vi "Step 2.vi"(8 "error in (no error)":errorcluster, 11 "HeatUp Data in":string[][](array[string])) -> (0 "error out":errorcluster, 1 "Large Draw":dbl[][](graph), 2 "Draw Flag":string[][](array[string]), 3 "Large Draw Flag Gallons":dbl)   [LabVIEW 2016]
uses:
  <vilib>/Utility/error.llb/DialogType.ctl
panel:
  out "Time":dbl
  # "Data with Stripped Header"
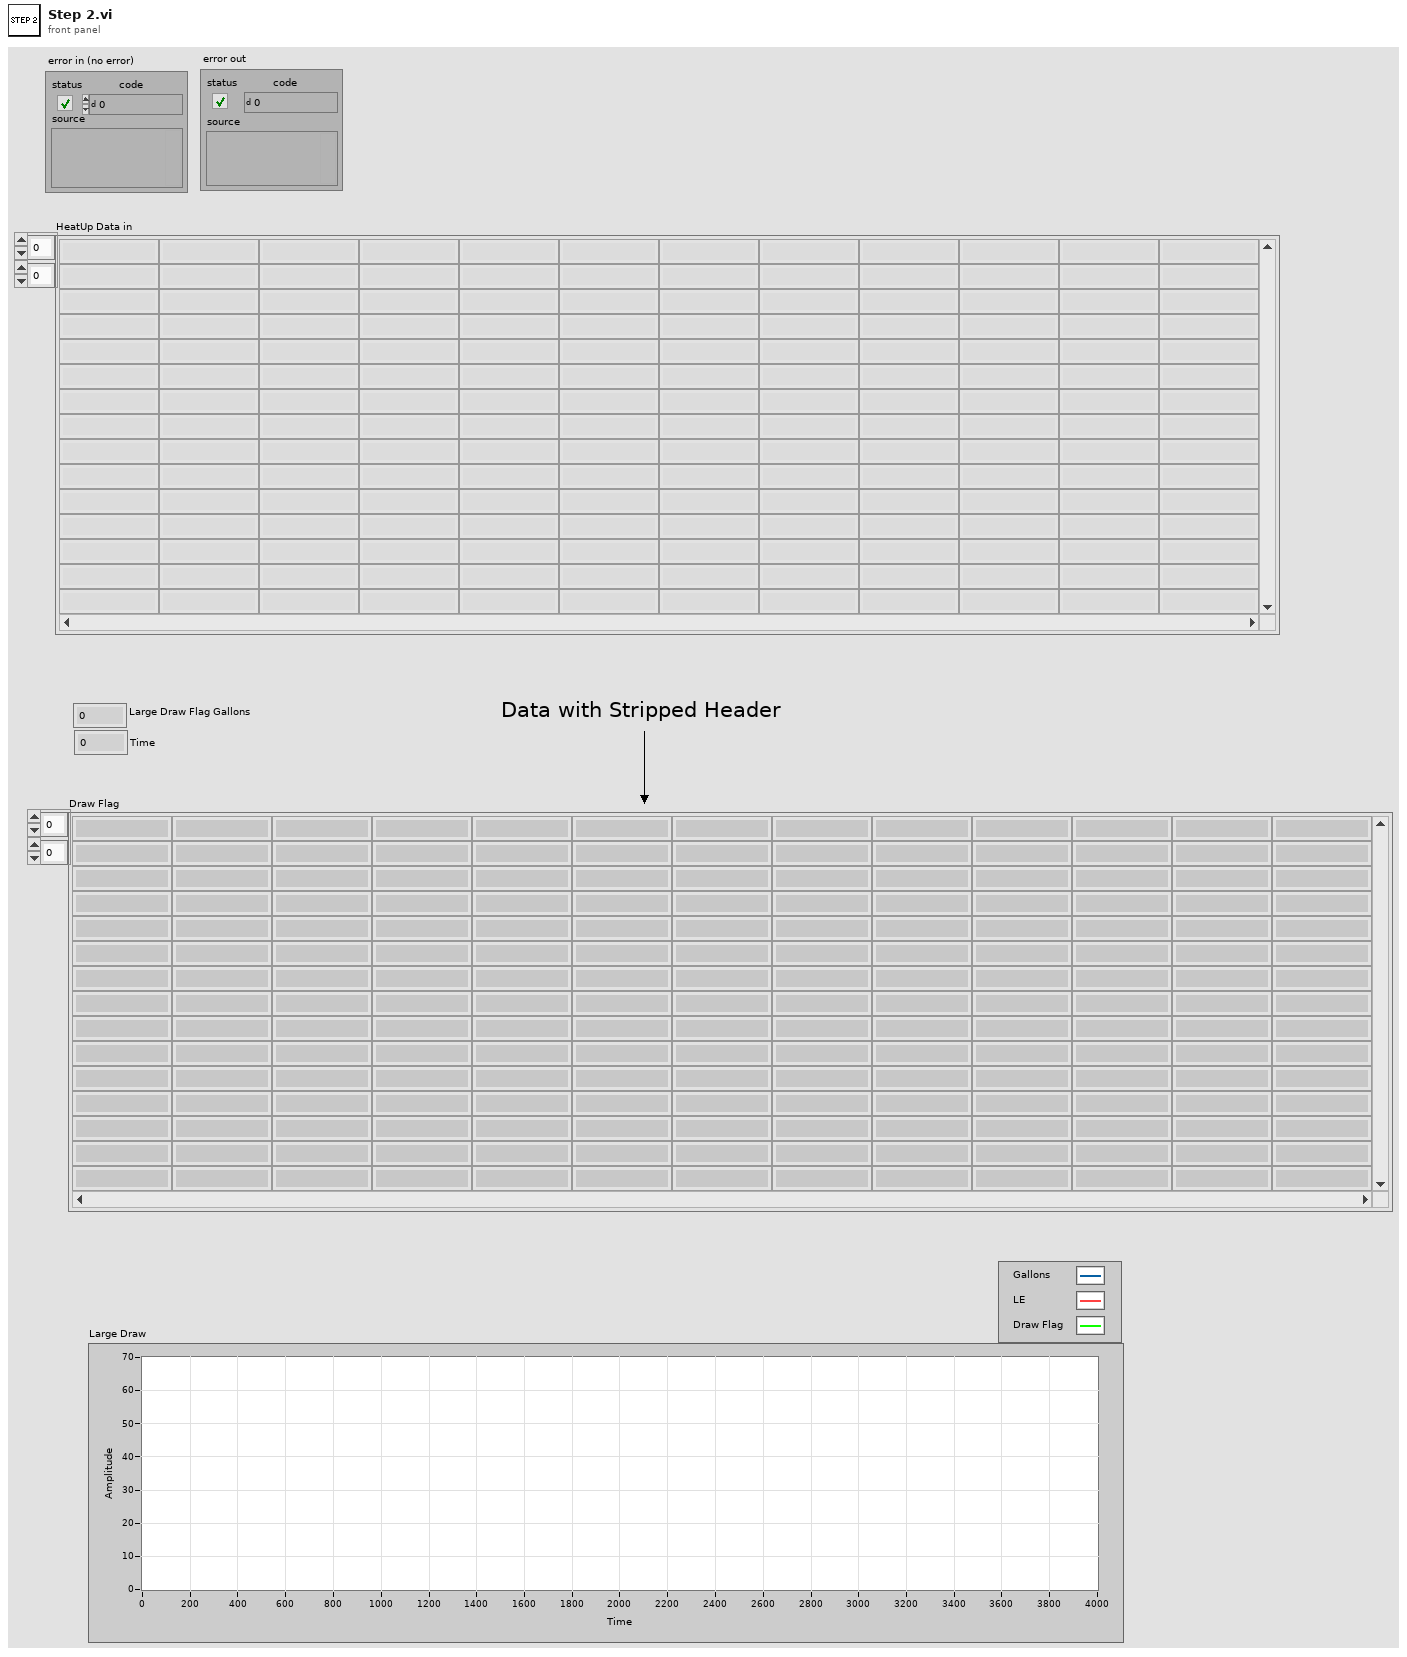
[diagram p1: front panel]
types:
  T1 = typedef "DialogType.ctl" = u16
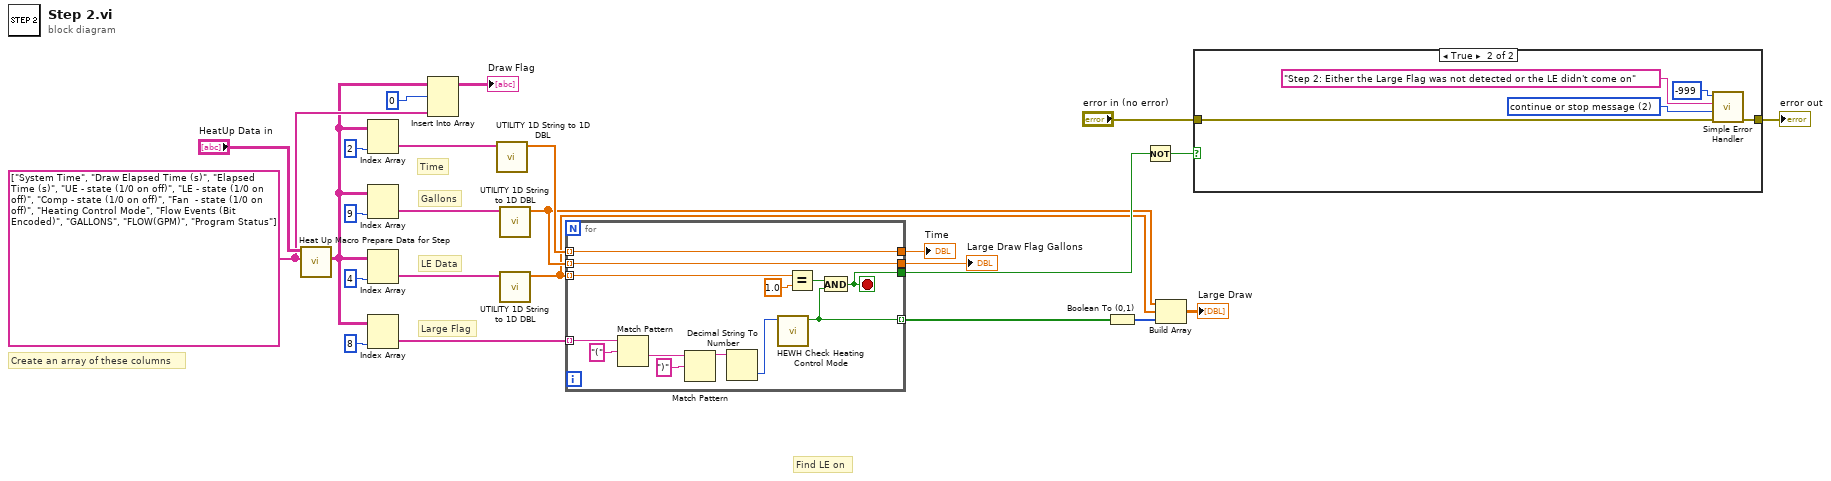
[diagram p0: block diagram]
diagram:
  w2 = string[] ["System Time", "Draw Elapsed Time (s)", "Elapsed Time (s)", "UE - state (1/0 on off)", "LE - state (1/0 on off)", "Comp - state (1/0 on off)", "Fan  - state (1/0 on off)", "Heating Control Mode", "Flow Events (Bit Encoded)", "GALLONS", "FLOW(GPM)", "Program Status"]
  # "Large Flag"
  # "LE Data"
  # "Time"
  # "Gallons"
  # "Find LE on"
  # "Create an array of these columns"
  n1 = call "Heat Up Macro Prepare Data for Step.vi"("Columns Too Search For"=w2, "HeatUp Raw Data Input"="HeatUp Data in") -> ("Heat Up Data with Only Selected Columns"=w1:string[][])  [unwired: 8 in, 1 out]
  n2 = Index Array(array=w1, index (col)=2 ("disabled index (col)")) -> (element=w21:string[])  [unwired: 1 in]
  n3 = Index Array(array=w1, index (col)=9 ("disabled index (col)")) -> (element=w22:string[])  [unwired: 1 in]
  n4 = Index Array(array=w1, index (col)=4 ("disabled index (col)")) -> (element=w23:string[])  [unwired: 1 in]
  n5 = Index Array(array=w1, index (col)=8 ("disabled index (col)")) -> (element=w15:string[])  [unwired: 1 in]
  n6 = Insert Into Array(array=w1, index (row)=0, new element=w2) -> (→"Draw Flag":string[][])  [unwired: 1 in]
  n7 = call "UTILITY 1D String to 1D DBL.vi"("Save Data"=w21) -> ("DBL"=w19:dbl[])  [unwired: 10 in]
  n8 = call "UTILITY 1D String to 1D DBL.vi"("Save Data"=w22) -> ("DBL"=w8:dbl[])  [unwired: 10 in]
  n9 = call "UTILITY 1D String to 1D DBL.vi"("Save Data"=w23) -> ("DBL"=w4:dbl[])  [unwired: 10 in]
  n10 = for {
    tunnel: w4 -> [w38] mode=indexing
    tunnel: w8 -> [w35] mode=indexing
    tunnel: w19 -> [w36] mode=indexing
    tunnel: [w36] -> w18
    tunnel: [w35] -> w17
    tunnel: w15 -> [w34] mode=indexing
    tunnel: [w27] -> w12
    tunnel: [w26] -> w7 mode=indexing
    stop <- w27 stop-if-true
    n11 = Match Pattern(string=w34, regular expression="(") -> (after substring=w32:string)  [unwired: 1 in, 3 out]
    n12 = Match Pattern(string=w32, regular expression=")") -> (before substring=w30:string)  [unwired: 1 in, 3 out]
    n13 = Decimal String To Number(string=w30) -> (number=w29:i32)  [unwired: 2 in, 1 out]
    n14 = call "HEWH Check Heating Control Mode.vi"("Flow Event"=w29) -> ("Large Flag Detected"=w26:bool)  [unwired: 10 in]
    n15 = Equal?(x=w38, y=1.0) -> (x = y?=w28:bool)
    n16 = And(x=w28, y=w26) -> (x .and. y?=w27:bool)
  }
  "Large Draw Flag Gallons" <- w17
  "Time" <- w18
  n17 = Boolean To (0,1)(Boolean=w7) -> (0, 1=w5:i16[])
  n18 = Not(x=w12) -> (.not. x?=w11:bool)
  n19 = Build Array(w8, w4, w5) -> (→"Large Draw":dbl[][])
  n20 = case shown="True" w11 {
    tunnel: "error in (no error)" -> [w39 w44]
    tunnel: [w39 w43] -> w13
    frame False {
    }
    frame True {
      w42 = T1 2 items=["no dialog", "OK message", "continue or stop message", "OK message + warnings", "continue/stop + warnings"] ("type of dialog (OK msg:1)")
      n21 = call <vilib>:"Simple Error Handler.vi"("error code (no error:0)"=-999, "error source (\" \")"="Step 2: Either the Large Flag was not detected or the LE didn't come on" ("error source (\" \")"), "type of dialog (OK msg:1)"=w42, "error in (no error)"=w44) -> ("error out"=w43:errorcluster)  [unwired: 1 in, 4 out]
    }
  }
  "error out" <- w13
